vi "Calc Currente Exposure Time.vi"(8 "error in (no error)":errorcluster, 11 "CCDCamera in":refnum<class "CCDCamera.lvclass">) -> (0 "error out":errorcluster, 3 "CCDCamera out":refnum<class "CCDCamera.lvclass">)   [LabVIEW 2018, in "CCDCamera.lvclass"]
uses:
  CCDCamera.lvclass
  C:/Users/observer/Desktop/SPARC4_ACS/SPARC4_ACS/Simulated_CCD_Camera/Simulated_CCD_Camera.lvclass
  Simulated_CCD_Camera/Simulated_CCD_Camera.lvclass/Simulated_CCD_Camera.ctl
  Interface/Interface.lvclass
  Simulated_CCD_Camera/Simulated_CCD_Camera.lvclass
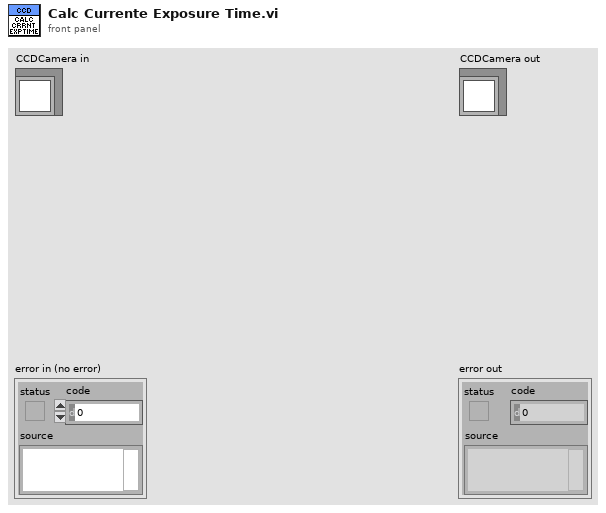
[diagram p1: front panel]
types:
  T1 = cluster{"CUBE_EXPOSURE_TIME":sgl, "CUBES_DONE":u16, "LAST_IMAGE_NAME":string, "DISK_SPACE":u16, "FRAMES_DONE":u16, "CCD_STATUS":string, "CURRENT_TEMPERATURE":i16, "TEMPERATURE_STATUS":string, "FRAME_EXPOSURE_TIME":u16, "CCD_ON_OFF":bool, "SERIAL_NUMBER":u16, "ACQUIRING":bool}
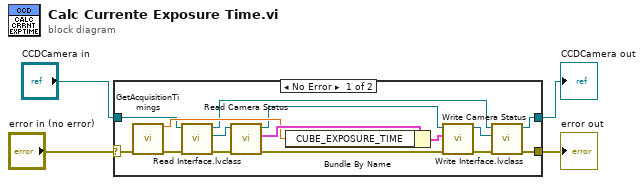
[diagram p0: block diagram]
diagram:
  n1 = case shown="No Error" "error in (no error)" {
    selector: "error in (no error)" -> [w19 w20]
    tunnel: "CCDCamera in" -> [w6 w21]
    tunnel: [w11 w20] -> w2
    tunnel: [w5 w21] -> w1
    frame No Error {
      n2 = call <userlib>:"GetAcquisitionTimings.vi"("error in (no error)"=w19) -> ("exposure"=w15:sgl, "error out"=w13:errorcluster)  [unwired: 10 in, 3 out]
      n3 = call "Read Interface.lvclass.vi"("error in (no error)"=w13, "Simulated_CCD_Camera in"=w6) -> ("error out"=w14:errorcluster, "Interface.lvclass"=w9:refnum<class "Interface.lvclass">, "Simulated_CCD_Camera out"=w10:refnum<class "CCDCamera.lvclass">)  [unwired: 7 in]
      n4 = call "Read Camera Status.vi"("error in (no error)"=w14, "Interface in"=w9) -> ("error out"=w16:errorcluster, "Camera Status"=w18:T1, "Interface out"=w7:refnum<class "Interface.lvclass">)  [unwired: 7 in]
      n5 = Bundle By Name(cluster=w18, "CUBE_EXPOSURE_TIME"=w15) -> (w17:T1)
      n6 = call "Write Camera Status.vi"("error in (no error)"=w16, "Camera Status"=w17, "Interface in"=w7) -> ("error out"=w12:errorcluster, "Interface out"=w8:refnum<class "Interface.lvclass">)  [unwired: 7 in]
      n7 = call "Write Interface.lvclass.vi"("error in (no error)"=w12, "Interface.lvclass"=w8, "Simulated_CCD_Camera in"=w10) -> ("error out"=w11:errorcluster, "Simulated_CCD_Camera out"=w5:refnum<class "CCDCamera.lvclass">)  [unwired: 7 in]
    }
    frame Error {
    }
  }
  "error out" <- w2
  "CCDCamera out" <- w1
